vi "LED Ctlr Sys Cal Factor.vi"() -> ()   [LabVIEW 2010]
uses:
  <vilib>/Analysis/NI_AALPro.lvlib
panel:
  out "error out":errorcluster
  out "Cal Factor":dbl
  out "Current Step":u16
  out "Max Illum LG":dbl caption="Gain_e" format="%.2f"
  out "Cal Factor LG":dbl caption="Gain_e" format="%.2g"
  out "Cal Factor HG":dbl caption="Gain_e" format="%.2g"
  out "Max Illum HG":dbl caption="Gain_e" format="%.2f"
  out "Calibration LG":cluster{dbl[], dbl[]}(graph)
  out "Calibration HG":cluster{dbl[], dbl[]}(graph)
  in  "OK":bool
  out "Status":string
  out "LG Cam Array":dbl[](array[numeric])
  out "HG Cam Array":dbl[](array[numeric])
  out "LG Det Array":dbl[](array[numeric])
  out "HG Det Array":dbl[](array[numeric])
  out "Illum % (Desired)":dbl
  out "Illum (Measured)":dbl format="%#_4g"
  in  "DAC Higher Limit":u32=5500
  in  "DAC Lower Limit":u32=300
  in  "Number of Steps":u32=21
  in  "Wavelength":string="1550"
  in  "LED Driver Com Port":refnum<visa-resource-name>="COM9"
  in  "Light Meter Port":refnum<visa-resource-name>="COM3"
  in  "error in (no error)":errorcluster
  # "Ver 1"
  # "AIS"
  # "Cal Factor Generator (LEDAD)"
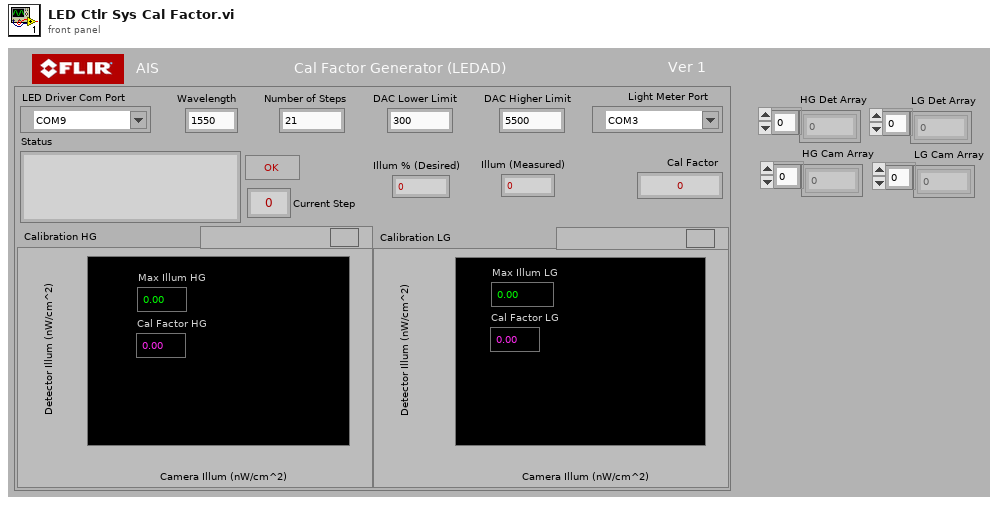
[diagram p1: front panel]
types:
  T1 = cluster{"HG Cam Array":dbl[], "HG Det Array":dbl[]}
  T2 = cluster{"LG Cam Array":dbl[], "LG Det Array":dbl[]}
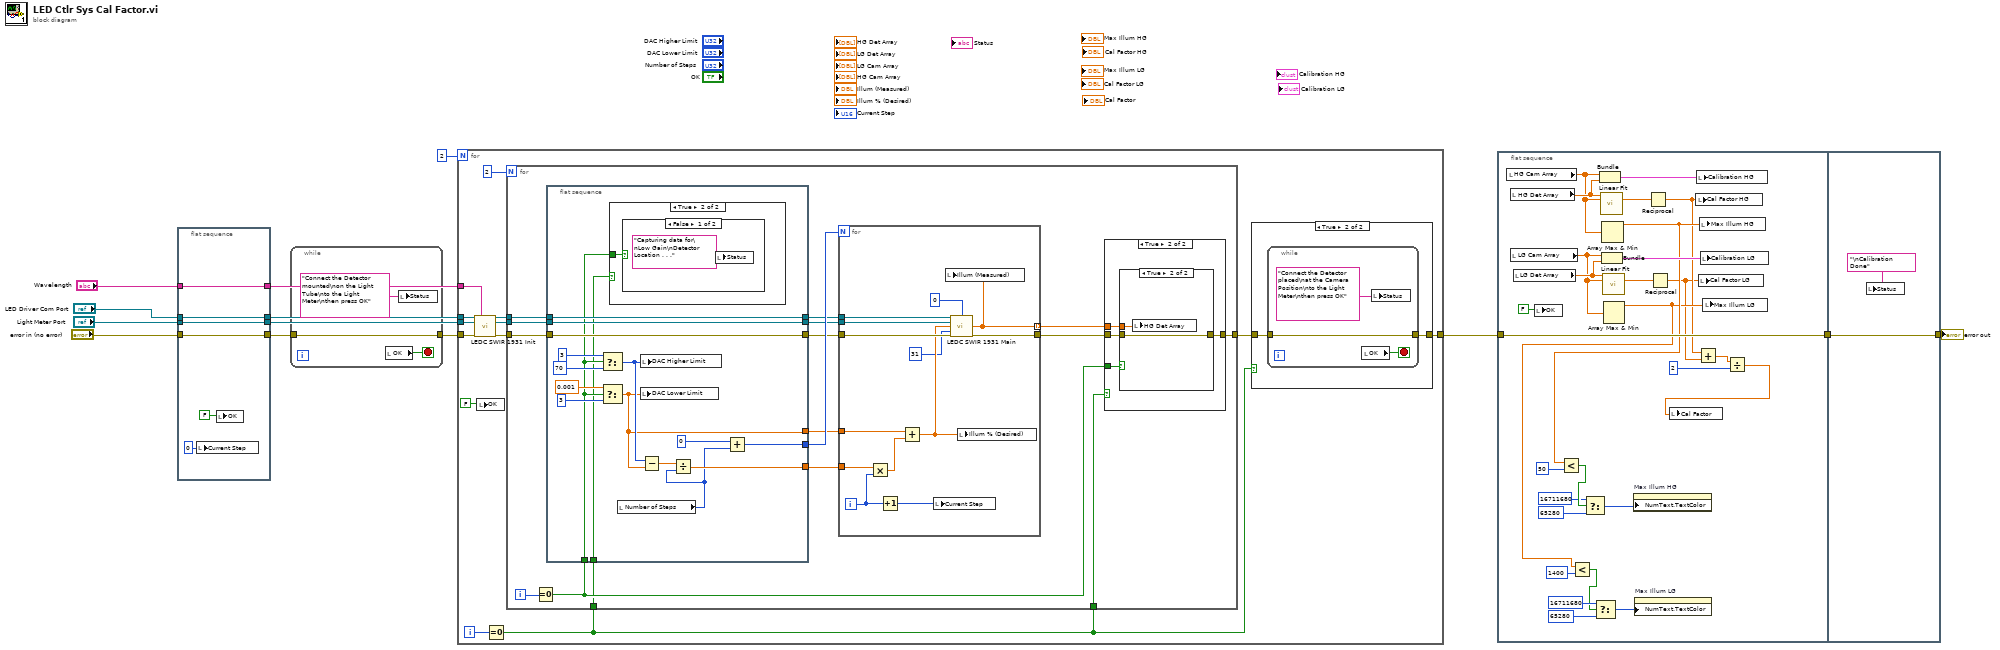
[diagram p0: block diagram]
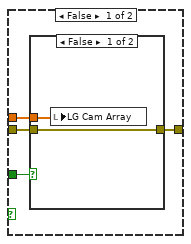
[diagram p3: hidden frame]
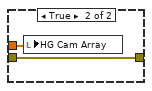
[diagram p4: hidden frame]
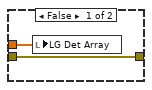
[diagram p5: hidden frame]
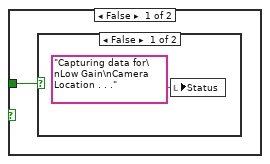
[diagram p6: hidden frame]
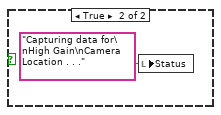
[diagram p7: hidden frame]
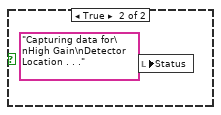
[diagram p8: hidden frame]
diagram:
  n1 = flat-sequence {
    tunnel: "Light Meter Port" -> [w16]
    tunnel: "LED Driver Com Port" -> [w17]
    tunnel: "Wavelength" -> [w14]
    tunnel: "error in (no error)" -> [w15]
    tunnel: [w17] -> w9
    tunnel: [w16] -> w8
    tunnel: [w15] -> w6
    tunnel: [w14] -> w1
    frame #0 {
      n2 = local write "Current Step"(0) -> ()
      n3 = local write "OK"(FALSE) -> ()
    }
  }
  n4 = while {
    tunnel: [w22] -> w5
    tunnel: w6 -> [w22]
    stop <- w20 stop-if-true
    n5 = local read "OK"() -> (w20:bool)
    n6 = local write "Status"("Connect the Detector mounted\non the Light Tube\nto the Light Meter\nthen press OK") -> ()
  }
  n7 = for {
    N: 2 -> [_]
    tunnel: w9 -> [w29]
    tunnel: w8 -> [w28]
    tunnel: w5 -> [w27]
    tunnel: [w33] -> w4
    tunnel: w1 -> [w23]
    i -> [w32]
    n8 = call "LEDC SWIR 1931 Init.vi"("LEDAD Port"=w29, "Wavelength"=w23, "Light Meter Port"=w28, "error in (no error)"=w27) -> ("LEDAD Port out"=w26:refnum<visa-resource-name>, "Light Meter Port out"=w25:refnum<visa-resource-name>, "error out"=w24:errorcluster)  [unwired: 7 in, 2 out]
    n9 = local write "OK"(FALSE) -> ()
    n10 = Equal To 0?(x=w32) -> (x = 0?=w30:bool)
    n11 = for {
      N: 2 -> [_]
      tunnel: w26 -> [w51]
      tunnel: w25 -> [w50]
      tunnel: w24 -> [w49]
      tunnel: [w44] -> w34
      tunnel: w30 -> [w43]
      tunnel: w30 -> [w42]
      i -> [w56]
      n12 = Equal To 0?(x=w56) -> (x = 0?=w55:bool)
      n13 = flat-sequence {
        tunnel: w55 -> [w77]
        tunnel: [w82] -> w54
        tunnel: [w81] -> w53
        tunnel: [w75] -> w52
        tunnel: [w80] -> w48
        tunnel: w51 -> [w80]
        tunnel: [w79] -> w47
        tunnel: w50 -> [w79]
        tunnel: [w78] -> w46
        tunnel: w49 -> [w78]
        tunnel: w42 -> [w76]
        frame #0 {
          n14 = Select(t=3, s=w77, f=70) -> (s? t:f=w83:i32)
          n15 = Select(t=0.001, s=w77, f=3) -> (s? t:f=w81:dbl)
          n16 = case shown="True" w76 {
            tunnel: w77 -> [w90 w93]
            frame False {
              n17 = case shown="False" w90 {
                frame False {
                  n18 = local write "Status"("Capturing data for\nLow Gain\nCamera Location . . .") -> ()
                }
                frame True {
                  n19 = local write "Status"("Capturing data for\nHigh Gain\nCamera Location . . .") -> ()
                }
              }
            }
            frame True {
              n20 = case shown="False" w93 {
                frame False {
                  n21 = local write "Status"("Capturing data for\nLow Gain\nDetector Location . . .") -> ()
                }
                frame True {
                  n22 = local write "Status"("Capturing data for\nHigh Gain\nDetector Location . . .") -> ()
                }
              }
            }
          }
          n23 = local read "Number of Steps"() -> (w74:u32)
          n24 = local write "DAC Lower Limit"(w81) -> ()
          n25 = local write "DAC Higher Limit"(w83) -> ()
          n26 = Subtract(x=w83, y=w81) -> (x-y=w88:dbl)
          n27 = Divide(x=w88, y=w74) -> (x/y=w75:dbl)
          n28 = Add(x=0, y=w74) -> (x+y=w82:u32)
        }
      }
      n29 = for {
        N: w54 -> [_]
        tunnel: w48 -> [w108]
        tunnel: w47 -> [w107]
        tunnel: w46 -> [w106]
        tunnel: w52 -> [w104]
        tunnel: w53 -> [w102]
        tunnel: [w100] -> w57 mode=indexing
        tunnel: [w99] -> w45
        i -> [w98]
        n30 = Multiply(x=w104, y=w98) -> (x*y=w103:dbl)
        n31 = Increment(x=w98) -> (x+1=w97:i32)
        n32 = Add(x=w102, y=w103) -> (x+y=w101:dbl)
        n33 = local write "Current Step"(w97) -> ()
        n34 = call "LEDC SWIR 1931 Main.vi"("LEDAD Port"=w108, "Unit"=0, "Light Meter Port"=w107, "Intensity Desired"=w101, "Enable LED"=31, "error in (no error)"=w106) -> ("Meas Illum"=w100:dbl, "error out"=w99:errorcluster)  [unwired: 4 in, 4 out]
        n35 = local write "Illum (Measured)"(w100) -> ()
        n36 = local write "Illum % (Desired)"(w101) -> ()
      }
      n37 = case shown="True" w43 {
        tunnel: w57 -> [w59 w69]
        tunnel: w55 -> [w58 w68]
        tunnel: w45 -> [w61 w67]
        tunnel: [w60 w66] -> w44
        frame False {
          n38 = case shown="False" w58 {
            tunnel: w59 -> [w63 w65]
            tunnel: [w62 w64] -> w60
            tunnel: w61 -> [w62 w64]
            frame False {
              n39 = local write "LG Cam Array"(w63) -> ()
            }
            frame True {
              n40 = local write "HG Cam Array"(w65) -> ()
            }
          }
        }
        frame True {
          n41 = case shown="True" w68 {
            tunnel: w69 -> [w71 w73]
            tunnel: [w70 w72] -> w66
            tunnel: w67 -> [w70 w72]
            frame False {
              n42 = local write "LG Det Array"(w71) -> ()
            }
            frame True {
              n43 = local write "HG Det Array"(w73) -> ()
            }
          }
        }
      }
    }
    n44 = case shown="True" w30 {
      tunnel: w34 -> [w36 w38]
      tunnel: [w36 w37] -> w33
      frame False {
      }
      frame True {
        n45 = while {
          tunnel: [w41] -> w37
          tunnel: w38 -> [w41]
          stop <- w39 stop-if-true
          n46 = local read "OK"() -> (w39:bool)
          n47 = local write "Status"("Connect the Detector placed\nat the Camera Position\nto the Light Meter\nthen press OK") -> ()
        }
      }
    }
  }
  n48 = flat-sequence {
    tunnel: w4 -> [w129]
    tunnel: [w129] -> w2
    tunnel: [w137] -> w3
    tunnel: w2 -> [w137]
    frame #0 {
      n49 = local read "HG Cam Array"() -> (w127:dbl[])
      n50 = local read "HG Det Array"() -> (w135:dbl[])
      n51 = local read "LG Cam Array"() -> (w126:dbl[])
      n52 = local read "LG Det Array"() -> (w132:dbl[])
      n53 = local write "OK"(FALSE) -> ()
      n54 = Bundle("HG Cam Array"=w127, "HG Det Array"=w135) -> (w134:T1)  [unwired: 1 in]
      n55 = call <vilib>:"Linear Fit.vi"("Y"=w135, "X"=w127) -> ("slope"=w112:dbl)  [unwired: 9 in, 4 out]
      n56 = Bundle("LG Cam Array"=w126, "LG Det Array"=w132) -> (w133:T2)  [unwired: 1 in]
      n57 = Array Max & Min(array=w127) -> (max value=w115:dbl)  [unwired: 3 out]
      n58 = Less?(x=w115, y=50) -> (x < y?=w125:bool)
      n59 = Select(t=u32 16711680, s=w125, f=u32 65280) -> (s? t:f=w121:u32)
      n60 = call <vilib>:"Linear Fit.vi"("Y"=w132, "X"=w126) -> ("slope"=w110:dbl)  [unwired: 9 in, 4 out]
      n61 = Array Max & Min(array=w126) -> (max value=w114:dbl)  [unwired: 3 out]
      n62 = Less?(x=w114, y=1400) -> (x < y?=w117:bool)
      n63 = Select(t=u32 16711680, s=w117, f=u32 65280) -> (s? t:f=w116:u32)
      n64 = property on="Max Illum HG" class="DigNum (strict)"("NumText.TextColor"=w121) -> ()  [unwired: 2 in, 2 out]
      n65 = property on="Max Illum LG" class="DigNum (strict)"("NumText.TextColor"=w116) -> ()  [unwired: 2 in, 2 out]
      n66 = Reciprocal(x=w112) -> (1/x=w111:dbl)
      n67 = Reciprocal(x=w110) -> (1/x=w109:dbl)
      n68 = local write "Cal Factor HG"(w111) -> ()
      n69 = local write "Calibration HG"(w134) -> ()
      n70 = Add(x=w111, y=w109) -> (x+y=w130:dbl)
      n71 = local write "Cal Factor LG"(w109) -> ()
      n72 = local write "Max Illum HG"(w115) -> ()
      n73 = local write "Calibration LG"(w133) -> ()
      n74 = local write "Max Illum LG"(w114) -> ()
      n75 = Divide(x=w130, y=2) -> (x/y=w128:dbl)
      n76 = local write "Cal Factor"(w128) -> ()
    }
    frame #1 {
      n77 = local write "Status"("\nCalibration Done") -> ()
    }
  }
  "error out" <- w3
